vi "FGV Variant.vi"(9 "Response to save":string, 10 "Command":string, 11 "Functions":enum16{"Reset data", "Set data", "Get data"}(ring)) -> (2 "Response retrieved":string, 3 "Variant":variant)   [LabVIEW 2020, in "Simulado.lvclass"]
uses:
  Simulado.lvclass
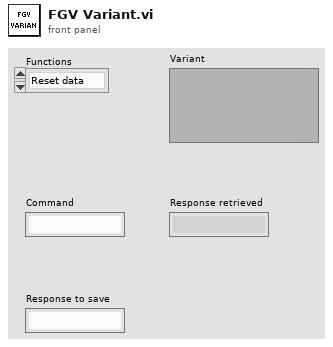
[diagram p1: front panel]
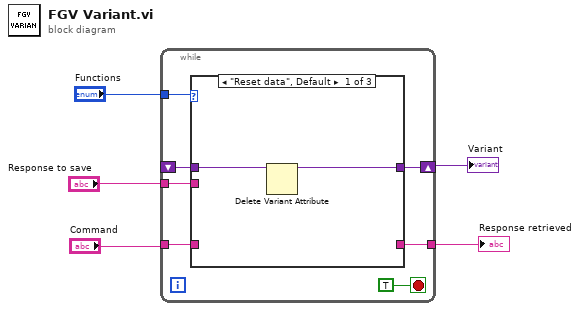
[diagram p0: block diagram]
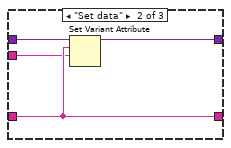
[diagram p2: hidden frame]
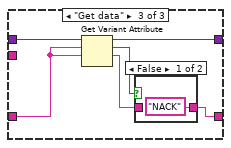
[diagram p3: hidden frame]
diagram:
  n1 = while {
    tunnel: "Functions" -> [w11]
    shift-right: [w9] -> w1
    shift-left: _ -> [w10]
    tunnel: "Command" -> [w8]
    tunnel: [w7] -> w4
    tunnel: "Response to save" -> [w6]
    stop <- TRUE stop-if-true
    n2 = case shown="\"Reset data\", Default" w11 {
      tunnel: w10 -> [w14 w18 w24]
      tunnel: [w13 w17 w23] -> w9
      tunnel: w8 -> [_ w16 w22]
      tunnel: [_ w16 w19] -> w7
      tunnel: w6 -> [_ w15 _]
      frame "Reset data", Default {
        n3 = Delete Variant Attribute(7:w14) -> (3:w13:variant)  [unwired: 2 in, 2 out]
      }
      frame "Set data" {
        n4 = Set Variant Attribute(Variant=w18, name=w16, value=w15) -> (Variant out=w17:variant)  [unwired: 1 in, 2 out]
      }
      frame "Get data" {
        n5 = Get Variant Attribute(Variant=w24, name=w22, default value (empty Variant)=w22) -> (duplicate Variant=w23:variant, found=w21:bool, value=w20:string)  [unwired: 1 in, 1 out]
        n6 = case shown="False" w21 {
          tunnel: w20 -> [_ w26]
          tunnel: ["NACK" ("Command") w26] -> w19
          frame False {
          }
          frame True {
          }
        }
      }
    }
  }
  "Variant" <- w1
  "Response retrieved" <- w4
